vi "Stand-alone Analysis.vi"   [LabVIEW 2020]
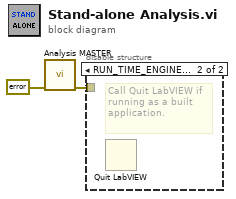
[diagram p0: block diagram]
diagram:
  n1 = call "Analysis MASTER.vi"("Error In"=errorcluster {"status"=FALSE, "code"=0, "source"=""}) -> ("Error Out"=w2:errorcluster)  [unwired: 10 in]
  n2 = disable-structure shown="RUN_TIME_ENGINE==True" {
    disable-tunnel: w2 -> [_ _]
    frame condition #0 (active) {
    }
    frame condition #1 {
      # "Call Quit LabVIEW if running as a built application."
      n3 = Quit LabVIEW() -> ()  [unwired: 1 in]
    }
  }
